vi "Main.vi"(8 "Error In":errorcluster, 10 "Folder":path=path "E:/LabVIEW/Data/Test Data/Subj-Austin_Trial-1_Condition-None.lvm" caption="Filename") -> (0 "Error Out":errorcluster)   [LabVIEW 2020]
uses:
  <vilib>/express/express shared/transition.llb/Dynamic To Waveform Array.vi
  <vilib>/express/express signal manip/GetorSetDDTAttributes/Shared VIs/XDimension conversion.vi
  <vilib>/express/express signal manip/GetorSetDDTAttributes/Shared VIs/XDimension Enum to String.vi
  <vilib>/express/express signal manip/GetorSetDDTAttributes/Shared VIs/TimeMode Enum to Boolean.vi
  <vilib>/express/express signal manip/GetorSetDDTAttributes/Set DDT Attributes/SetT0.vi
  <vilib>/express/express signal manip/GetorSetDDTAttributes/Set DDT Attributes/sub Set StartTimeStamp.vi
  <vilib>/express/express shared/transition.llb/Waveform Array To Dynamic.vi
  <vilib>/express/express signal manip/GetorSetDDTAttributes/Get DDT Attributes/Get DDT Properties.xnode
  <vilib>/express/express signal manip/GetorSetDDTAttributes/Shared VIs/TimeType.ctl
  <vilib>/express/express signal manip/GetorSetDDTAttributes/Shared VIs/XDimension.ctl
  <vilib>/express/express signal manip/GetorSetDDTAttributes/Set DDT Attributes/Set DDT Properties.xnode
  <vilib>/express/express signal manip/GetorSetDDTAttributes/Shared VIs/GetSetShared.lvlib
  <vilib>/express/express signal manip/GetorSetDDTAttributes/Set DDT Attributes/Set DDT Attributes.lvlib
panel:
  out "Total Rows Deleted":i32
  out "Display Table":string[][](table)
  out "Progress Bar":u8(slide) max=10 scale=0.9..27.0
  out "Number of Files Found":i32
  in  "Stop Button":bool
  out "Files Checked":i32
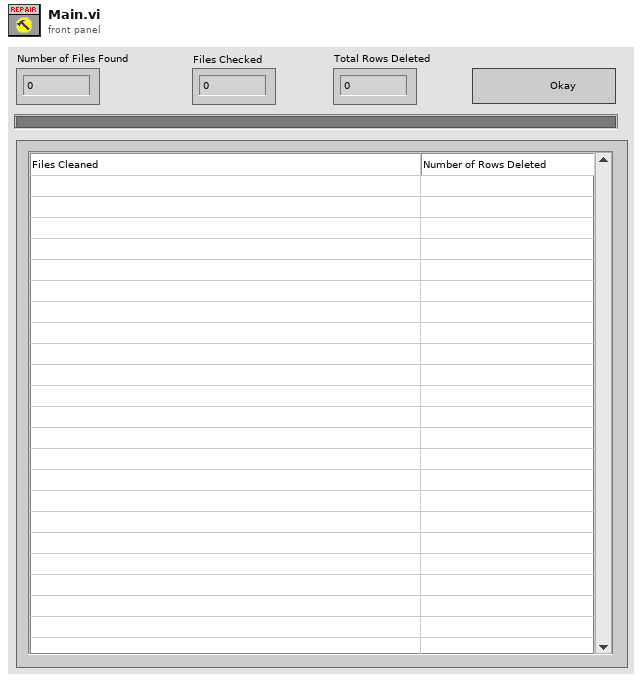
[diagram p1: front panel]
types:
  T1 = typedef "GetSetShared.lvlib/TimeType.ctl" = enum16{"Absolute", "Relative"}
  T2 = typedef "GetSetShared.lvlib/XDimension.ctl" = enum16{"No Unit [-]", "Time [sec]", "Frequency [Hz]"}
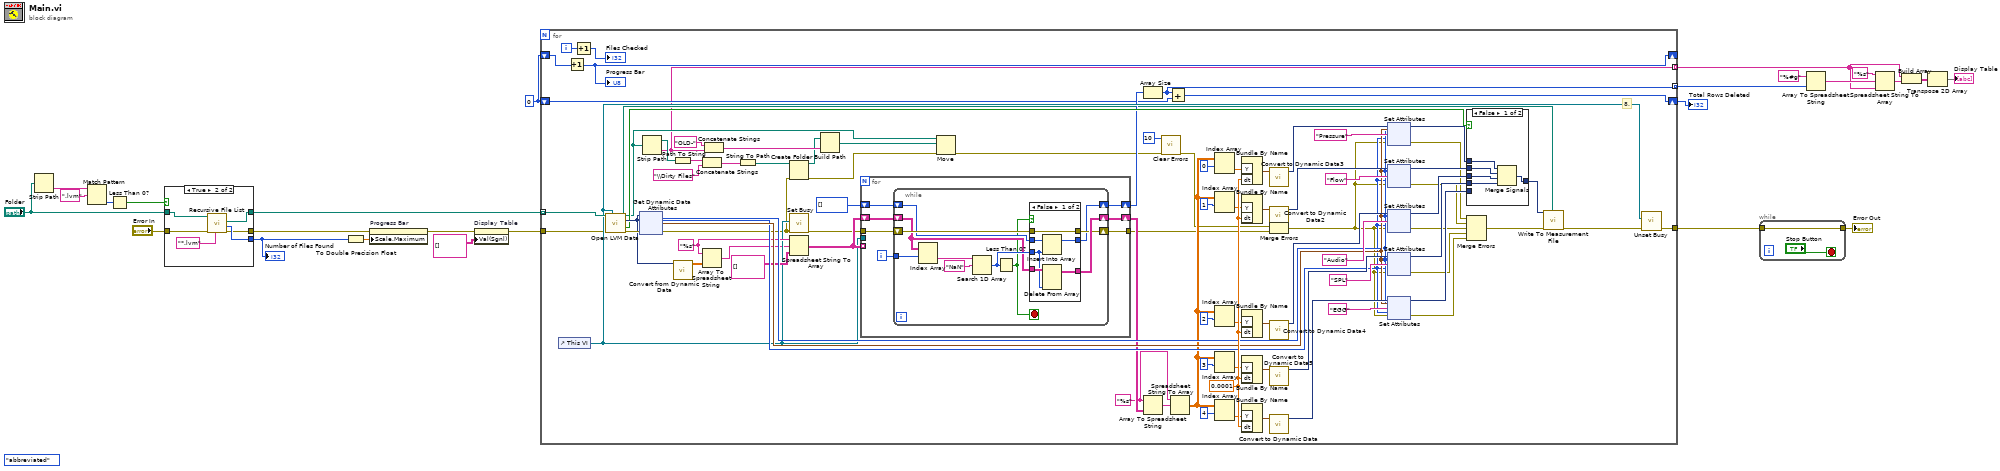
[diagram p0: block diagram]
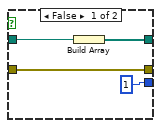
[diagram p2: hidden frame]
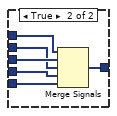
[diagram p4: hidden frame]
diagram:
  (unwired) enum16{"short", "long", "abbreviated"}."abbreviated" ("date format (0)")
  w2 = 0 ("x+1")
  n1 = Strip Path(path="Folder") -> (name=w10:string)  [unwired: 1 out]
  n2 = Match Pattern(string=w10, regular expression=".lvm") -> (offset past match=w8:i32)  [unwired: 1 in, 3 out]
  n3 = Less Than 0?(x=w8) -> (x < 0?=w7:bool)
  n4 = case shown="True" w7 {
    tunnel: "Error In" -> [w27 w35]
    tunnel: [w28 w33] -> w24
    tunnel: [1 ("Number of Files") w32] -> w16
    tunnel: [w27 w31] -> w14
    tunnel: "Folder" -> [w29 w30]
    frame False {
      n5 = Build Array(w29) -> (w28:path[])
    }
    frame True {
      n6 = call <vilib>:"Recursive File List.vi"("pattern"="*.lvm", "error in (no error)"=w35, "Folder Path"=w30) -> ("error out"=w31:errorcluster, "Number of Files"=w32:i32, "All Files in Dir"=w33:path[])  [unwired: 4 in, 2 out]
    }
  }
  "Number of Files Found" <- w16
  n7 = To Double Precision Float(number=w16) -> (double precision float=w15:dbl)
  n8 = property on="Progress Bar" class="Slide (strict)"(error in=w14, "Scale.Maximum"=w15) -> (error out=w5:errorcluster)  [unwired: 1 in, 1 out]
  n9 = property on="Display Table" class="Tbl (strict)"(error in=w5, "Val(Sgnl)"=string[][] [] ("Value (Signaling)")) -> (error out=w4:errorcluster)  [unwired: 1 in, 1 out]
  n10 = for {
    tunnel: w4 -> [w45]
    tunnel: [w100] -> w22
    tunnel: w24 -> [w64] mode=indexing
    tunnel: [w39] -> w18 mode=indexing
    tunnel: [w57] -> w17 mode=indexing
    shift-right: [w60] -> _
    shift-left: w2 -> [w61]
    shift-right: [w56] -> w1
    shift-left: w2 -> [w58]
    i -> [w66]
    w76 = "%s" ("format string")
    w81 = "%s" ("format string")
    w101 = 0.0001 ("dt")
    # "8."
    n11 = control-ref of="This VI"() -> (w63:refnum<vi>)
    n12 = Increment(x=w61) -> (x+1=w60:i32)
    "Progress Bar" <- w60
    n13 = Increment(x=w66) -> (x+1=→"Files Checked":i32)
    n14 = call "Open LVM Data.vi"("Filename"=w64, "VI reference"=w63, "Error In"=w45) -> ("Filename Out"=w47:path, "All Data"=w82:dynamicdata, "EGG?"=w69:bool, "Error Out"=w88:errorcluster)  [unwired: 9 in]
    n15 = xnode "Get Dynamic Data Attributes"("Signals In"=w82, "error in"=w88) -> ("error out"=w44:errorcluster, "Time Mode"=w85:T1, "Timestamp"=w87:timestamp, "X Dimension"=w86:T2)  [unwired: 1 in, 2 out]
    n16 = Strip Path(path=w47) -> (stripped path=w54:path, name=w39:string)
    n17 = Path To String(path=w54) -> (string=w53:string)
    n18 = call "Convert from Dynamic Data"("Dynamic Data Type"=w82) -> ("Array"=w79:dbl[][])  [unwired: 3 in]
    n19 = Concatenate Strings(w53, "\\Dirty Files" ("string")) -> (w51:string)
    n20 = Array To Spreadsheet String(array=w79, 3:w81) -> (spreadsheet string=w48:string)  [unwired: 1 in]
    n21 = Concatenate Strings("OLD-" ("string"), w39) -> (w43:string)
    n22 = String To Path(string=w51) -> (path=w42:path)
    n23 = Create Folder(path (use dialog)=w42, error in=w44) -> (created path=w41:path, error out=w38:errorcluster)  [unwired: 1 in, 1 out]
    n24 = call <vilib>:"Set Busy.vi"("error in (no error)"=w44, "VI reference (current VI)"=w63) -> ("error out"=w62:errorcluster)  [unwired: 8 in, 1 out]
    n25 = Spreadsheet String To Array(format string=w81, spreadsheet string=w48, array type (2D Dbl)=string[][] []) -> (array=w68:string[][])  [unwired: 1 in]
    n26 = Build Path(base path=w41, name or relative path=w43) -> (appended path=w46:path)
    n27 = for {
      tunnel: [w125] -> w50
      tunnel: w62 -> [w124]
      shift-right: [w126] -> w59
      shift-left: i32[] [] -> [w127]
      tunnel: w63 -> [_]
      shift-right: [w128] -> w77
      shift-left: w68 -> [w123]
      tunnel: w68 -> [_] mode=indexing
      i -> [w122]
      n28 = while {
        shift-right: [w137] -> w128
        shift-left: w123 -> [w131]
        shift-right: [w135] -> w125
        shift-left: w124 -> [w136]
        shift-right: [w133] -> w126
        shift-left: w127 -> [w134]
        tunnel: w122 -> [w132]
        stop <- w129 stop-if-true
        n29 = Index Array(array=w131, index (row)=w132) -> (element=w130:string[])  [unwired: 1 in]
        n30 = Search 1D Array(1D array=w130, element="NaN") -> (index of element=w138:i32)  [unwired: 1 in]
        n31 = Less Than 0?(x=w138) -> (x < 0?=w129:bool)
        n32 = case shown="False" w129 {
          tunnel: w138 -> [w140 _]
          tunnel: [w145 w148] -> w137
          tunnel: w131 -> [w144 w148]
          tunnel: w136 -> [w143 w147]
          tunnel: [w143 w147] -> w135
          tunnel: w134 -> [w142 w146]
          tunnel: [w141 w146] -> w133
          frame False {
            n33 = Insert Into Array(array=w142, new element=w140) -> (w141:i32[])  [unwired: 1 in]
            n34 = Delete From Array(array=w144, index (col)=w140) -> (array with subset deleted=w145:string[][])  [unwired: 2 in, 1 out]
          }
          frame True {
          }
        }
      }
    }
    n35 = Move(source path=w47, error in=w38, 10:w46) -> (error out=w37:errorcluster)  [unwired: 2 in, 2 out]
    n36 = Array Size(array=w59) -> (size(s)=w57:i32)
    n37 = Array To Spreadsheet String(array=w77, 3:w76) -> (spreadsheet string=w75:string)  [unwired: 1 in]
    n38 = call <vilib>:"Clear Errors.vi"("error in (no error)"=w37, "specific error code to clear (0: all)"=10) -> ("error out"=w36:errorcluster)  [unwired: 4 in, 1 out]
    n39 = Add(x=w57, y=w58) -> (x+y=w56:i32)
    n40 = Spreadsheet String To Array(format string=w76, spreadsheet string=w75) -> (array=w78:dbl[][])  [unwired: 2 in]
    n41 = Index Array(array=w78, index (row)=0) -> (element=w74:dbl[])  [unwired: 1 in]
    n42 = Index Array(array=w78, index (row)=1) -> (element=w73:dbl[])  [unwired: 1 in]
    n43 = Index Array(array=w78, index (row)=2) -> (element=w72:dbl[])  [unwired: 1 in]
    n44 = Index Array(array=w78, index (row)=3) -> (element=w71:dbl[])  [unwired: 1 in]
    n45 = Index Array(array=w78, index (row)=4) -> (element=w70:dbl[])  [unwired: 1 in]
    n46 = Bundle By Name("Y"=w74, "dt"=w101) -> (w106:waveform(dbl))  [unwired: 1 in]
    n47 = Bundle By Name("Y"=w73, "dt"=w101) -> (w105:waveform(dbl))  [unwired: 1 in]
    n48 = Bundle By Name("Y"=w72, "dt"=w101) -> (w102:waveform(dbl))  [unwired: 1 in]
    n49 = Bundle By Name("Y"=w71, "dt"=w101) -> (w103:waveform(dbl))  [unwired: 1 in]
    n50 = Bundle By Name("Y"=w70, "dt"=w101) -> (w104:waveform(dbl))  [unwired: 1 in]
    n51 = call "Convert to Dynamic Data3"("Waveform"=w106) -> ("Dynamic Data Type"=w118:dynamicdata)  [unwired: 3 in]
    n52 = call "Convert to Dynamic Data2"("Waveform"=w105) -> ("Dynamic Data Type"=w116:dynamicdata)  [unwired: 3 in]
    n53 = Merge Errors(w36, w50) -> (w49:errorcluster)
    n54 = call "Convert to Dynamic Data4"("Waveform"=w102) -> ("Dynamic Data Type"=w113:dynamicdata)  [unwired: 3 in]
    n55 = call "Convert to Dynamic Data5"("Waveform"=w103) -> ("Dynamic Data Type"=w111:dynamicdata)  [unwired: 3 in]
    n56 = call "Convert to Dynamic Data"("Waveform"=w104) -> ("Dynamic Data Type"=w110:dynamicdata)  [unwired: 3 in]
    n57 = xnode "Set Attributes"("Signals In"=w118, "error in"=w49, "Signal Name"="Pressure", "Time Mode"=w85, "Timestamp"=w87, "X Dimension"=w86) -> ("Signals Out"=w107:dynamicdata, "error out"=w93:errorcluster)  [unwired: 2 in]
    n58 = xnode "Set Attributes"("Signals In"=w116, "error in"=w49, "Signal Name"="Flow", "Time Mode"=w85, "Timestamp"=w87, "X Dimension"=w86) -> ("Signals Out"=w114:dynamicdata, "error out"=w92:errorcluster)  [unwired: 2 in]
    n59 = xnode "Set Attributes"("Signals In"=w113, "error in"=w49, "Signal Name"="Audio", "Time Mode"=w85, "Timestamp"=w87, "X Dimension"=w86) -> ("Signals Out"=w112:dynamicdata, "error out"=w91:errorcluster)  [unwired: 2 in]
    n60 = xnode "Set Attributes"("Signals In"=w111, "error in"=w49, "Signal Name"="SPL", "Time Mode"=w85, "Timestamp"=w87, "X Dimension"=w86) -> ("Signals Out"=w109:dynamicdata, "error out"=w90:errorcluster)  [unwired: 2 in]
    n61 = xnode "Set Attributes"("Signals In"=w110, "error in"=w49, "Signal Name"="EGG", "Time Mode"=w85, "Timestamp"=w87, "X Dimension"=w86) -> ("Signals Out"=w108:dynamicdata, "error out"=w89:errorcluster)  [unwired: 2 in]
    n62 = case shown="False" w69 {
      tunnel: [w334 w340] -> w84
      tunnel: w107 -> [w333 w339]
      tunnel: w114 -> [w332 w337]
      tunnel: w112 -> [w331 w338]
      tunnel: w109 -> [w330 w336]
      tunnel: w108 -> [_ w335]
      frame False {
        n63 = Merge Signals(w333, w332, w331, w330) -> (w334:dynamicdata)
      }
      frame True {
        n64 = Merge Signals(w339, w338, w337, w336, w335) -> (w340:dynamicdata)
      }
    }
    n65 = Merge Errors(w93, w92, w91, w90, w89) -> (w94:errorcluster)
    n66 = call "Write To Measurement File"("Signals"=w84, "error in (no error)"=w94, "Filename"=w47) -> ("error out"=w67:errorcluster)  [unwired: 14 in, 2 out]
    n67 = call <vilib>:"Unset Busy.vi"("error in (no error)"=w67, "VI reference (current VI)"=w63) -> ("error out"=w100:errorcluster)  [unwired: 9 in]
  }
  "Total Rows Deleted" <- w1
  n68 = while {
    tunnel: w22 -> [w341]
    tunnel: [w341] -> w12
    stop <- "Stop Button" stop-if-true
  }
  "Error Out" <- w12
  n69 = Array To Spreadsheet String(array=w17, 3:"%#g" ("format string")) -> (spreadsheet string=w19:string)  [unwired: 1 in]
  n70 = Spreadsheet String To Array(format string="%s", spreadsheet string=w19, array type (2D Dbl)=w18) -> (array=w20:string[])  [unwired: 1 in]
  n71 = Build Array(w18, w20) -> (w21:string[][])
  n72 = Transpose 2D Array(2D array=w21) -> (transposed array=→"Display Table":string[][])
